vi "Sensor Simulation Main Page.vi"(8 "error in (no error)":errorcluster, 11 "Node Ptr":T1 format="%.0x") -> (0 "error out":errorcluster)   [LabVIEW 2010, in "Sensor Simulation Custom Device.lvlib"]
uses:
  Sensor Simulation Custom Device.lvlib
  <vilib>/NI VeriStand/Custom Device API/Custom Device Item Ref.ctl
  Global.vi
  <vilib>/NI VeriStand/Custom Device API/Get Item Property (Boolean).vi
  <vilib>/NI VeriStand/Custom Device API/Get Item Property (String).vi
  <vilib>/NI VeriStand/Custom Device API/Get Item Property (Dependent File).vi
  <vilib>/NI VeriStand/Custom Device API/Get Item Property (Dependent Node Pointer).vi
  <vilib>/NI VeriStand/Custom Device API/Set Item Property (String).vi
  <vilib>/NI Veristand/Custom Device API/Custom Device API.lvlib
  <userlib>/_FPGA Interface Advanced Tools/FPGA Bitfile Utility/FPGA Bitfile Utility.lvlib
panel:
  in  "SHDocVw.IWebBrowser2":refnum<k7>(container)
  out "Original Checksum":string
  out "Current Checksum":string
  in  "FPGA Name":string
  in  "Name":string
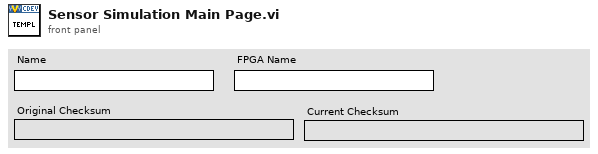
[diagram p1: front panel]
types:
  T1 = typedef "Custom Device API.lvlib/Custom Device Item Ref.ctl" = u64
  T2 = typedef "Custom Device API.lvlib/Custom Device Item Info.ctl" = cluster{"Name":string, "Is Channel":bool, "GUID":string}
  T3 = typedef "Custom Device API.lvlib/Custom Device Commands.ctl" = enum16{"Default", "Item renamed", "Shutdown", "Dynamic button pressed"}
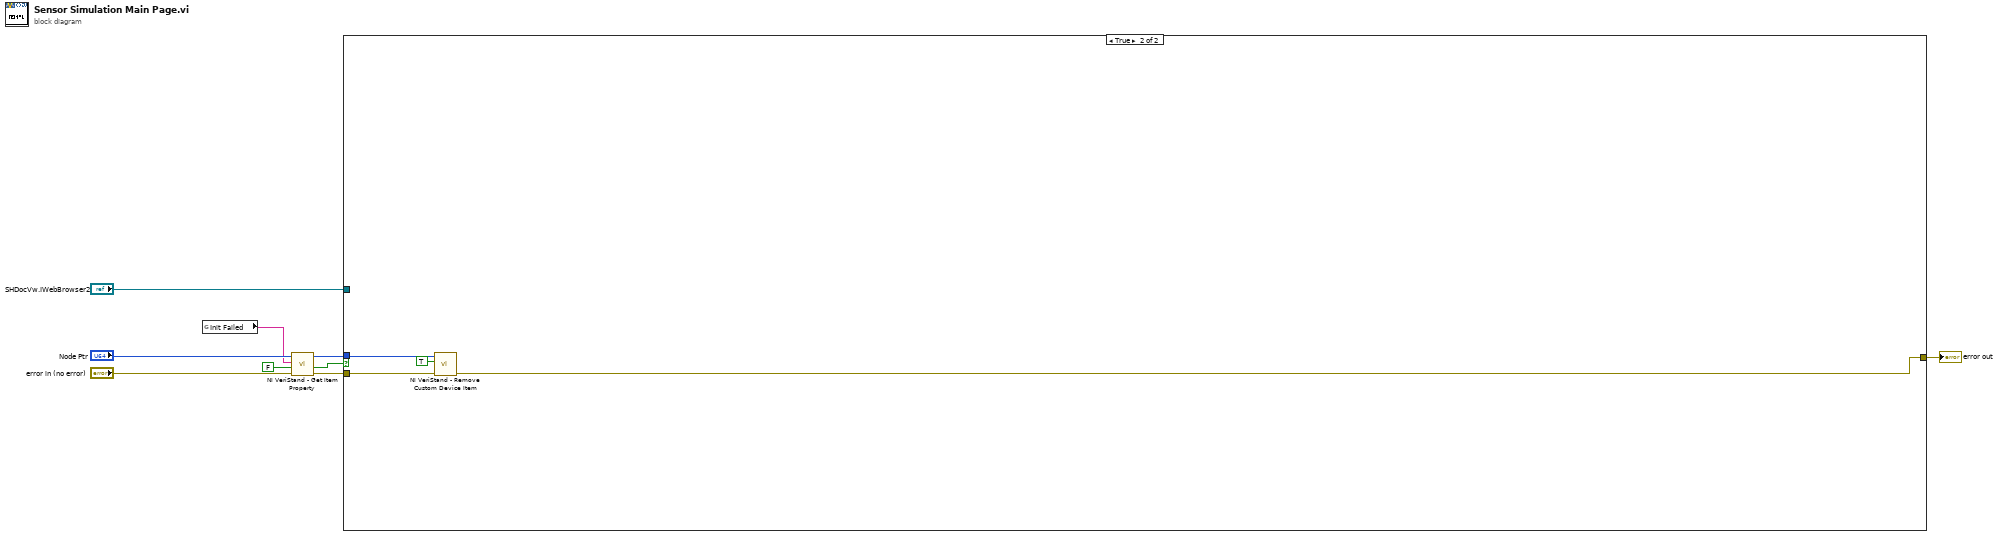
[diagram p0: block diagram]
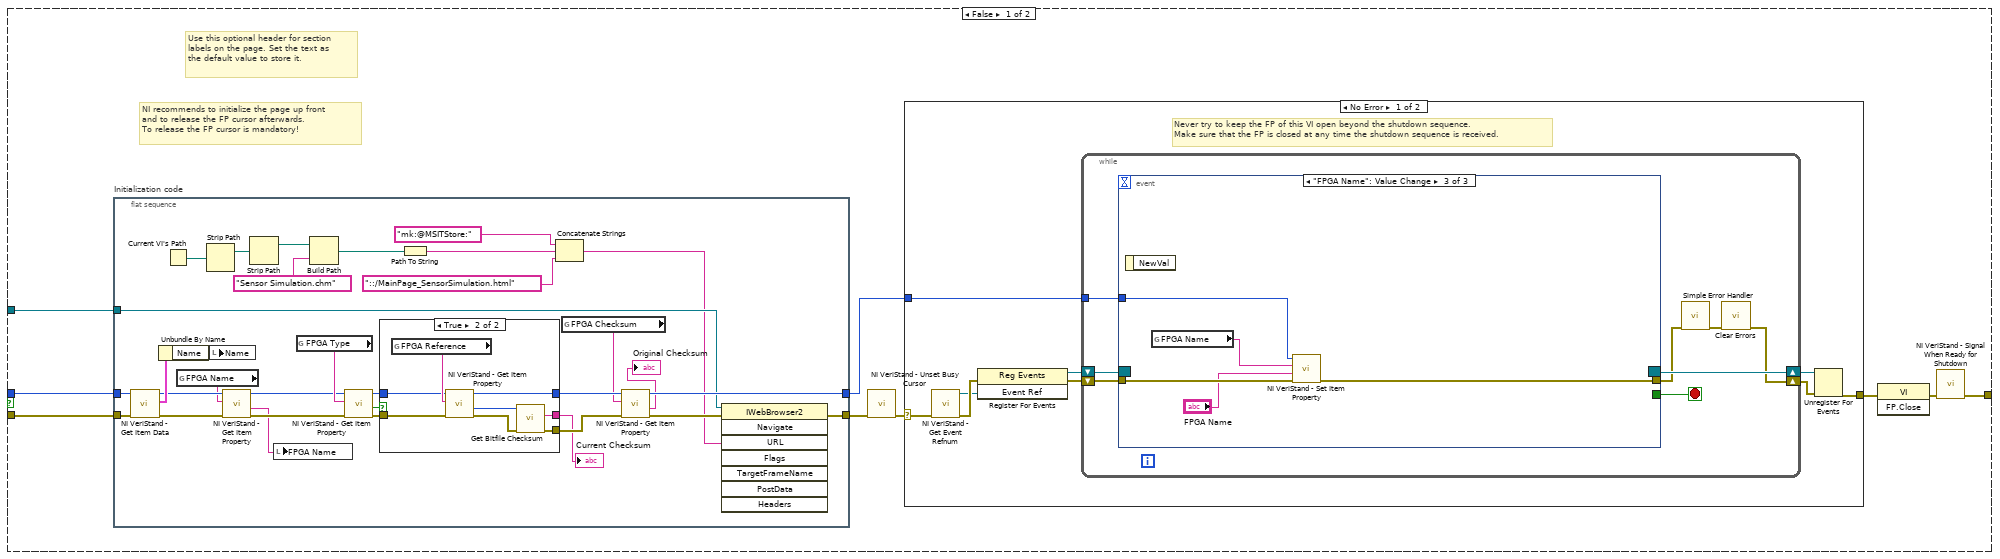
[diagram p2: hidden frame]
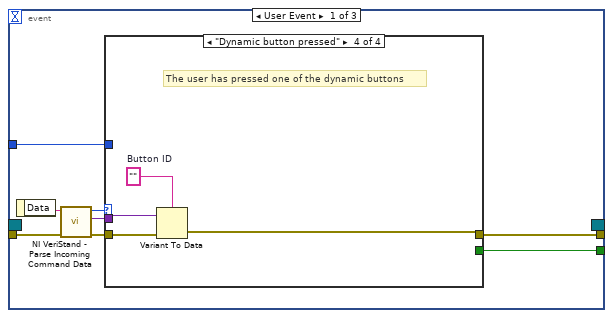
[diagram p3: hidden frame]
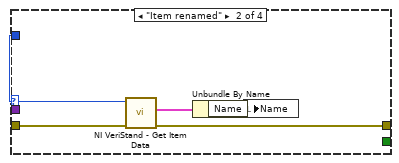
[diagram p5: hidden frame]
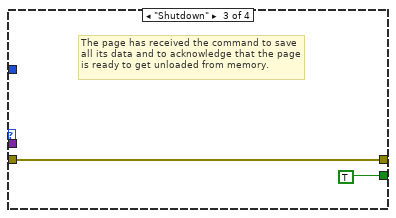
[diagram p6: hidden frame]
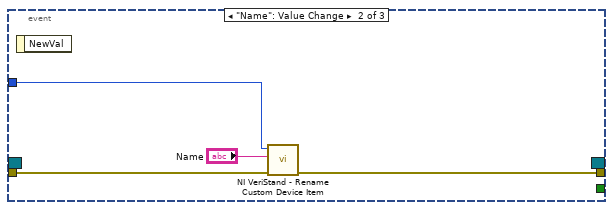
[diagram p7: hidden frame]
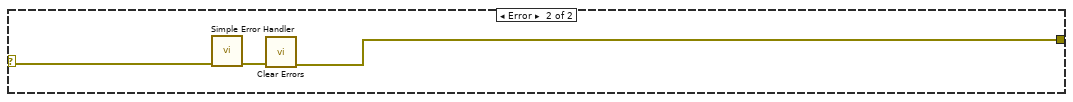
[diagram p8: hidden frame]
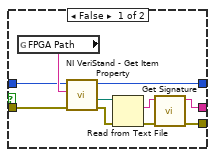
[diagram p9: hidden frame]
diagram:
  n1 = global read "Global.vi" "Init Failed"() -> (w4:string)
  n2 = call-poly <vilib>:"NI VeriStand - Get Item Property.vi"("error in (no error)"="error in (no error)", "Default Value"=FALSE, "Property Name"=w4, "Item Ref in"="Node Ptr") -> ("error out"=w7:errorcluster, "Value"=w2:bool, "Item Ref out"=w5:T1)  [unwired: 4 in, 1 out]
  n3 = case shown="True" w2 {
    tunnel: [w16 w119] -> w9
    tunnel: w5 -> [w15 w120]
    tunnel: w7 -> [w10 w118]
    tunnel: "SHDocVw.IWebBrowser2" -> [w11 _]
    frame False {
      # "Use this optional header for section labels on the page. Set the text as the default value to store it."
      # "NI recommends to initialize the page up front\nand to release the FP cursor afterwards.\nTo release the FP cursor is mandatory!"
      n4 = flat-sequence "Initialization code" {
        tunnel: w10 -> [w81]
        tunnel: w15 -> [w82]
        tunnel: [w70] -> w14
        tunnel: [w91] -> w12
        tunnel: w11 -> [w71]
        frame #0 {
          n5 = call <vilib>:"NI VeriStand - Get Item Data.vi"("error in (no error)"=w81, "Item Ref in"=w82) -> ("error out"=w97:errorcluster, "Item Info"=w99:T2, "Item Ref out"=w96:T1)  [unwired: 7 out]
          n6 = Unbundle By Name(w99) -> ("Name"=w98:string)
          n7 = Current VI's Path() -> (path=w79:path)
          n8 = global read "Global.vi" "FPGA Name"() -> (w95:string)
          n9 = Strip Path(path=w79) -> (stripped path=w78:path)  [unwired: 1 out]
          n10 = local write "Name"(w98) -> ()
          n11 = call-poly <vilib>:"NI VeriStand - Get Item Property.vi"("error in (no error)"=w97, "Property Name"=w95, "Item Ref in"=w96) -> ("error out"=w86:errorcluster, "Value"=w68:string, "Item Ref out"=w87:T1)  [unwired: 5 in, 1 out]
          n12 = Strip Path(path=w78) -> (stripped path=w73:path)  [unwired: 1 out]
          n13 = local write "FPGA Name"(w68) -> ()
          n14 = global read "Global.vi" "FPGA Type"() -> (w88:string)
          n15 = Build Path(base path=w73, name or relative path="Sensor Simulation.chm") -> (appended path=w75:path)
          n16 = call-poly <vilib>:"NI VeriStand - Get Item Property.vi"("error in (no error)"=w86, "Property Name"=w88, "Item Ref in"=w87) -> ("error out"=w83:errorcluster, "Value"=w85:bool, "Item Ref out"=w84:T1)  [unwired: 5 in, 1 out]
          n17 = case shown="True" w85 {
            tunnel: [w100 w117] -> w94
            tunnel: [w106 w113] -> w93
            tunnel: [w105 w112] -> w90
            tunnel: w84 -> [w108 w111]
            tunnel: w83 -> [w107 w110]
            frame False {
              n18 = global read "Global.vi" "FPGA Path"() -> (w109:string)
              n19 = call-poly <vilib>:"NI VeriStand - Get Item Property.vi"("error in (no error)"=w107, "Property Name"=w109, "Item Ref in"=w108) -> ("error out"=w104:errorcluster, "Path"=w102:path, "Item Ref out"=w100:T1)  [unwired: 4 in, 2 out]
              n20 = Read from Text File(file (use dialog)=w102, error in=w104) -> (text=w103:string, error out=w101:errorcluster)  [unwired: 2 in, 2 out]
              n21 = call <userlib>:"Get Signature.vi"("error in (no error)"=w101, "bitfile xml in"=w103) -> ("error out"=w106:errorcluster, "Bitfile Signature"=w105:string)  [unwired: 7 in, 1 out]
            }
            frame True {
              n22 = global read "Global.vi" "FPGA Reference"() -> (w116:string)
              n23 = call-poly <vilib>:"NI VeriStand - Get Item Property.vi"("error in (no error)"=w110, "Property Name"=w116, "Item Ref in"=w111) -> ("error out"=w114:errorcluster, "Dependent Node Ref"=w115:T1, "Item Ref out"=w117:T1)  [unwired: 5 in, 1 out]
              n24 = call "Get Bitfile Checksum.vi"("error in (no error)"=w114, "ID in"=w115) -> ("error out"=w113:errorcluster, "MD5"=w112:string)  [unwired: 6 in, 2 out]
            }
          }
          "Current Checksum" <- w90
          n25 = Path To String(path=w75) -> (string=w76:string)
          n26 = Concatenate Strings("mk:@MSITStore:" ("string"), w76, "::/MainPage_SensorSimulation.html" ("name or relative path")) -> (w69:string)
          n27 = global read "Global.vi" "FPGA Checksum"() -> (w92:string)
          n28 = call-poly <vilib>:"NI VeriStand - Get Item Property.vi"("error in (no error)"=w93, "Property Name"=w92, "Item Ref in"=w94) -> ("error out"=w72:errorcluster, "Value"=→"Original Checksum":string, "Item Ref out"=w91:T1)  [unwired: 5 in, 1 out]
          n29 = invoke class="IWebBrowser2" method="Navigate"(reference=w71, error in=w72, "URL"=w69) -> (error out=w70:errorcluster)  [unwired: 5 in, 7 out]
        }
      }
      n30 = call <vilib>:"NI VeriStand - Unset Busy Cursor.vi"("error in (no error)"=w14) -> ("error out"=w13:errorcluster)  [unwired: 10 out]
      n31 = case shown="No Error" w13 {
        selector: w13 -> [w19 w67]
        tunnel: [w24 w65] -> w18
        tunnel: w12 -> [w20 _]
        frame No Error {
          # "Never try to keep the FP of this VI open beyond the shutdown sequence.\nMake sure that the FP is closed at any time the shutdown sequence is received."
          n32 = call <vilib>:"NI VeriStand - Get Event Refnum.vi"("error in (no error)"=w19) -> ("error out"=w27:errorcluster, "Event Ref"=w23:refnum<user-event>)  [unwired: 9 out]
          n33 = register-events(error in=w27, w23) -> (reference out=w21:refnum<event-registration>, error out=w22:errorcluster)  [unwired: 1 in]
          n34 = while {
            tunnel: w20 -> [w31]
            shift-right: [w28] -> w25
            shift-left: w22 -> [w34]
            shift-right: [w35] -> w26
            shift-left: w21 -> [w33]
            stop <- w32 stop-if-true
            n35 = event shown="[2] \"FPGA Name\": Value Change" {
              selector: w33 -> [_ _ _]
              dyn-events: [_ _ _] -> w35
              timeout: _ -> [_ _ _]
              tunnel: w34 -> [w43 w59 w64]
              tunnel: [w39 _ _] -> w32
              tunnel: [w38 w58 w60] -> w30
              tunnel: w31 -> [w37 w57 w63]
              event User Event {
                n36 = event-data() -> ("Data"=w42:string)  [unwired: 1 out]
                n37 = call <vilib>:"NI VeriStand - Parse Incoming Command Data.vi"("error in (no error)"=w43, "Data"=w42) -> ("error out"=w41:errorcluster, "Data"=w36:variant, "Action"=w40:T3)  [unwired: 7 out]
                n38 = case shown="\"Dynamic button pressed\"" w40 {
                  tunnel: w41 -> [w44 w49 w50 w55]
                  tunnel: [_ _ TRUE _] -> w39
                  tunnel: [w44 w46 w50 w52] -> w38
                  tunnel: w37 -> [_ w48 _ _]
                  tunnel: w36 -> [_ _ _ w54]
                  frame "Default", Default {
                  }
                  frame "Item renamed" {
                    n39 = call <vilib>:"NI VeriStand - Get Item Data.vi"("error in (no error)"=w49, "Item Ref in"=w48) -> ("error out"=w46:errorcluster, "Item Info"=w47:T2)  [unwired: 8 out]
                    n40 = Unbundle By Name(w47) -> ("Name"=w45:string)
                    n41 = local write "Name"(w45) -> ()
                  }
                  frame "Shutdown" {
                    # "The page has received the command to save all its data and to acknowledge that the page is ready to get unloaded from memory."
                  }
                  frame "Dynamic button pressed" {
                    w53 = ""  # Button ID
                    # "The user has pressed one of the dynamic buttons"
                    n42 = Variant To Data(error in=w55, Variant=w54, type=w53) -> (error out=w52:errorcluster)  [unwired: 1 out]
                  }
                }
              }
              event "Name": Value Change {
                n43 = event-data() -> ()  [unwired: 2 out]
                n44 = call <vilib>:"NI VeriStand - Rename Custom Device Item.vi"("error in (no error)"=w59, "New Name"="Name", "Item Ref in"=w57) -> ("error out"=w58:errorcluster)  [unwired: 8 out]
              }
              event "FPGA Name": Value Change {
                n45 = event-data() -> ()  [unwired: 2 out]
                n46 = global read "Global.vi" "FPGA Name"() -> (w61:string)
                n47 = call-poly <vilib>:"NI VeriStand - Set Item Property.vi"("error in (no error)"=w64, "Value"="FPGA Name", "Property Name"=w61, "Item Ref in"=w63) -> ("error out"=w60:errorcluster)  [unwired: 5 in, 2 out]
              }
            }
            n48 = call <vilib>:"Simple Error Handler.vi"("error in (no error)"=w30) -> ("error out"=w29:errorcluster)  [unwired: 1 in, 7 out]
            n49 = call <vilib>:"Clear Errors.vi"("error in (no error)"=w29) -> ("error out"=w28:errorcluster)  [unwired: 6 out]
          }
          n50 = Unregister For Events(event registration refnum=w26, error in=w25) -> (error out=w24:errorcluster)
        }
        frame Error {
          n51 = call <vilib>:"Simple Error Handler.vi"("error in (no error)"=w67) -> ("error out"=w66:errorcluster)  [unwired: 1 in, 7 out]
          n52 = call <vilib>:"Clear Errors.vi"("error in (no error)"=w66) -> ("error out"=w65:errorcluster)  [unwired: 6 out]
        }
      }
      n53 = invoke class="VI" method="FP.Close"(error in=w18) -> (error out=w17:errorcluster)  [unwired: 2 in, 2 out]
      n54 = call <vilib>:"NI VeriStand - Signal When Ready for Shutdown.vi"("error in (no error)"=w17) -> ("error out"=w16:errorcluster)  [unwired: 10 out]
    }
    frame True {
      n55 = call <vilib>:"NI VeriStand - Remove Custom Device Item.vi"("error in (no error)"=w118, "Force Delete (F)"=TRUE, "Item Ref in"=w120) -> ("error out"=w119:errorcluster)  [unwired: 7 in, 1 out]
    }
  }
  "error out" <- w9
